vi "Set Enable Debugging.vi"(8 "error in (no error)":errorcluster, 9 "Wait for debugger on launch (false)":bool, 10 "Enable debugging (false)":bool, 11 "PPL in":refnum<class "NI_AB_API_PPL.lvclass">) -> (0 "error out":errorcluster, 3 "PPL out":refnum<class "NI_AB_API_PPL.lvclass">)   [LabVIEW 2020, in "NI_AB_API_PPL.lvclass"]
uses:
  <vilib>/AppBuilder/AB_API/PPL/NI_AB_API_PPL.lvclass
  <vilib>/AppBuilder/AB_API/Targetfile/NI_AB_API_Targetfile.lvclass
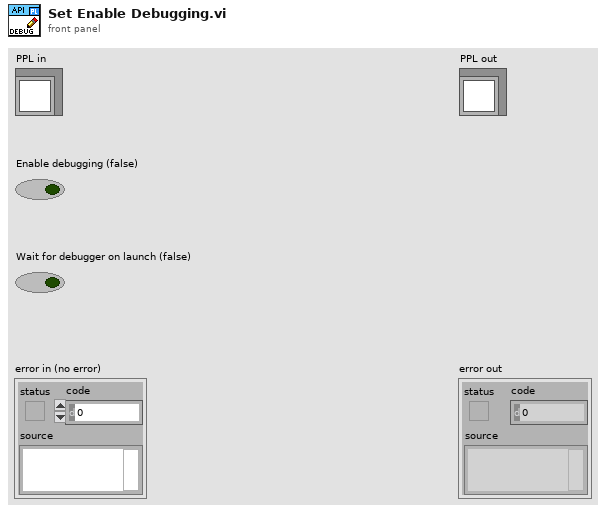
[diagram p1: front panel]
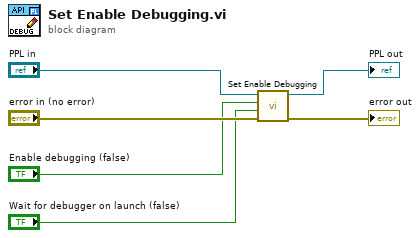
[diagram p0: block diagram]
diagram:
  n1 = call-parent "Set Enable Debugging.vi"("error in (no error)"="error in (no error)", "Wait for debugger on launch (false)"="Wait for debugger on launch (false)", "Enable debugging (false)"="Enable debugging (false)", "NI_AB_API_Targetfile in"="PPL in") -> ("error out"=→"error out":errorcluster, "NI_AB_API_Targetfile out"=→"PPL out":refnum<class "NI_AB_API_PPL.lvclass">)  [unwired: 6 in]
